vi "ZDataVIS_Offset+Multiplier.vi"(11 "Vfast":dbl[](array[numeric])) -> (3 "Cluster":cluster{dbl, dbl})   [LabVIEW 2016]
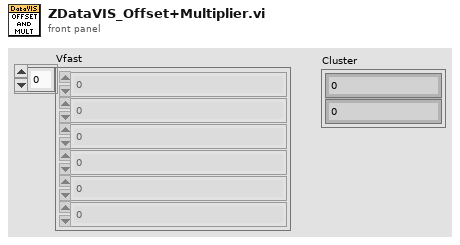
[diagram p1: front panel]
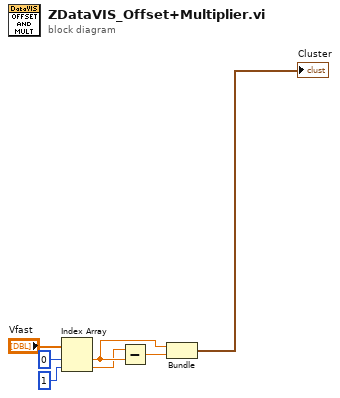
[diagram p0: block diagram]
diagram:
  n1 = Index Array(array="Vfast", index #1=0 ("index"), index #2=1 ("index")) -> (element #1=w7:dbl, element #2=w3:dbl)
  n2 = Subtract(x=w3, y=w7) -> (x-y=w6:dbl)
  n3 = Bundle(w7, w6) -> (→"Cluster":cluster{dbl, dbl})  [unwired: 1 in]
